vi "CRYView Model LIB.vi"(7 "sAction":string, 8 "nData":i32, 9 "sData":string, 10 "sOption":string, 11 "cView":T1) -> (0 "nData_Out":i32, 1 "sData_Out":string, 3 "cView_Out":T1)   [LabVIEW 2013]
uses:
  CRYView Global.vi
  CRYCurveLibrary/Global/CRYCurve Library Global.vi
  CRYNew View Global.vi
panel:
  out "pSPRef_Out":refnum<vi>
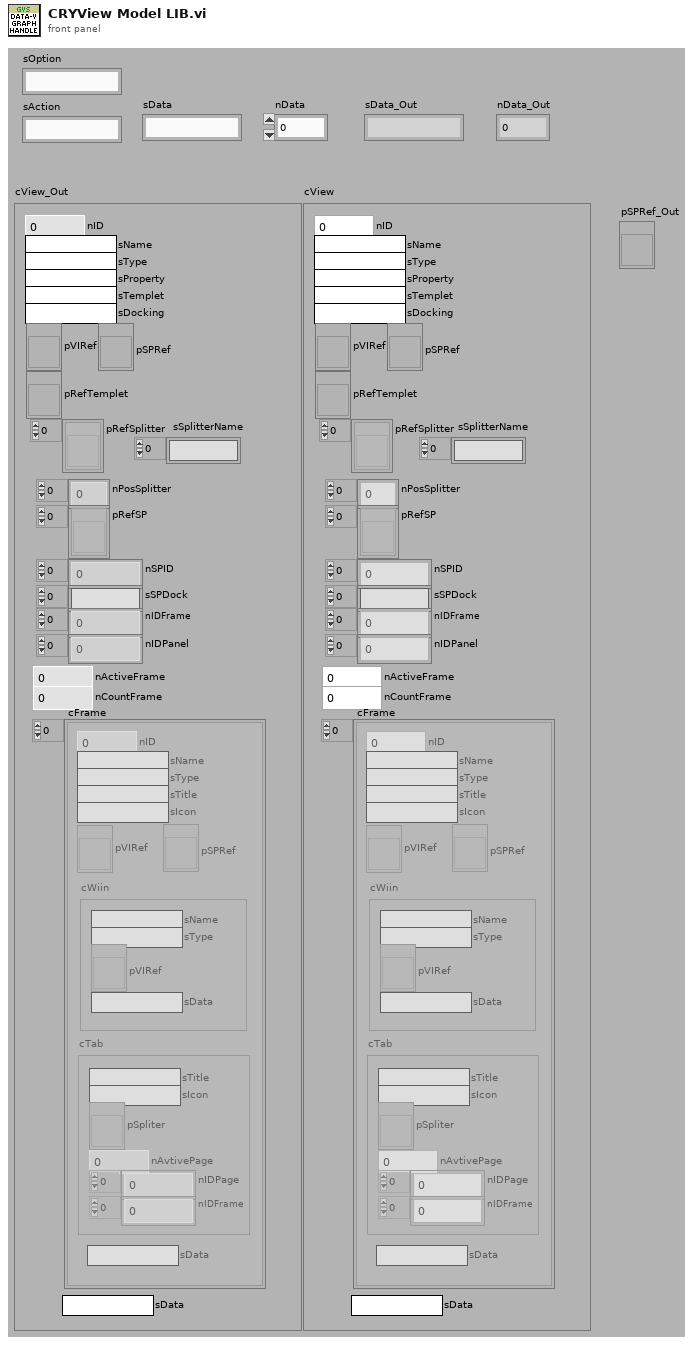
[diagram p1: front panel]
types:
  T1 = cluster{"nID":i32, "sName":string, "sType":string, "sProperty":string, "sTemplet":string, "sDocking":string, "pVIRef":refnum<vi>, "pSPRef":refnum<vi>, "pRefTemplet":refnum<vi>, "pRefSplitter":refnum<vi>[], "nPosSplitter":i32[], "pRefSP":refnum<vi>[], "nSPID":i32[], "sSPDock":string[], "nIDFrame":i32[], "nIDPanel":i32[], "nActiveFrame":i32, "nCountFrame":i32, "cFrame":cluster{"nID":i32, "sName":string, "sType":string, "sTitle":string, "sIcon":string, "pVIRef":refnum<vi>, "pSPRef":refnum<vi>, "cWiin":cluster{"sName":string, "sType":string, "pVIRef":refnum<vi>, "sData":string}, "cTab":cluster{"sTitle":string, "sIcon":string, "pSpliter":refnum<vi>, "nAvtivePage":i32, "nIDPage":i32[], "nIDFrame":i32[]}, "sData":string}[], "sData":string, "sSplitterName":string[]}
  T2 = typedef "Graph Main Info Cluster.ctl" = cluster{"Selected_BarIdx":i32, "Selected_PanelIdx":i32, "Graph Main VIRef":refnum<vi>, "ToolBarClick":bool, "Spliter Ref Array":refnum<vi>[], "Panel Ref Array":refnum<vi>[], "Spliter_matrix":i32[][], "Panel_matrix":i32[][], "child_spliterIdx_matrix":i32[][], "split_pos_matrix":i32[][], "Title State":bool, "sQueueName":string, "Frame nID":i32, "Graph VIRef Array":cluster{"Graph VIRef":refnum<vi>, "Panel Idx":i32, "Frame VIRef":refnum<vi>, "Icon Ring":i32, "Graph Type":string}[], "View Type":string}
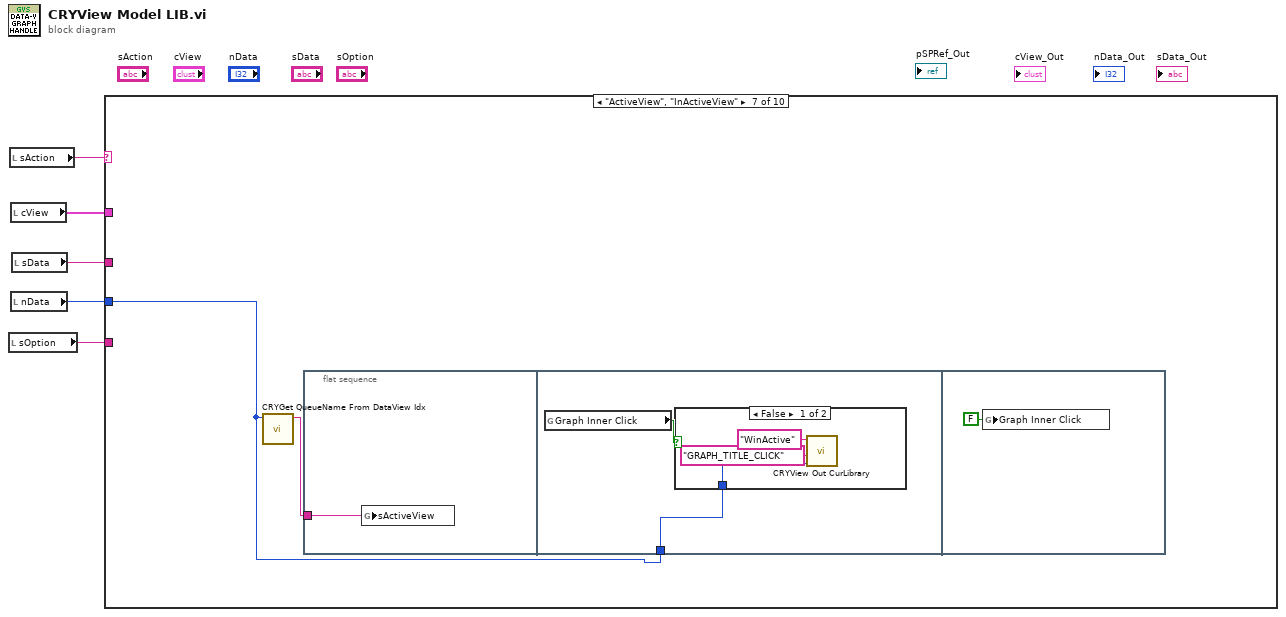
[diagram p0: block diagram]
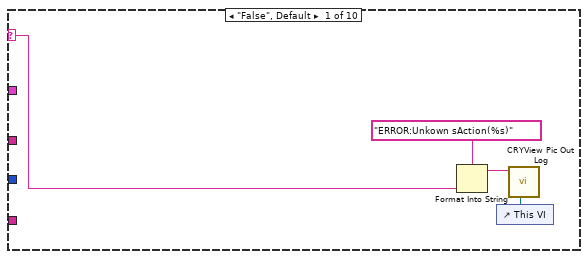
[diagram p2: hidden frame]
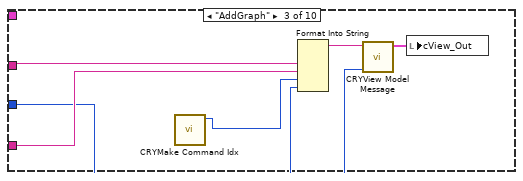
[diagram p4: hidden frame]
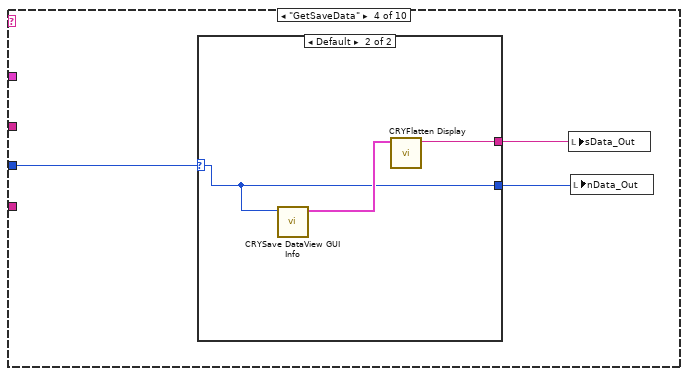
[diagram p5: hidden frame]
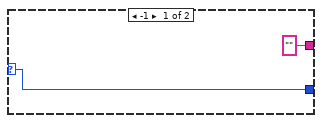
[diagram p6: hidden frame]
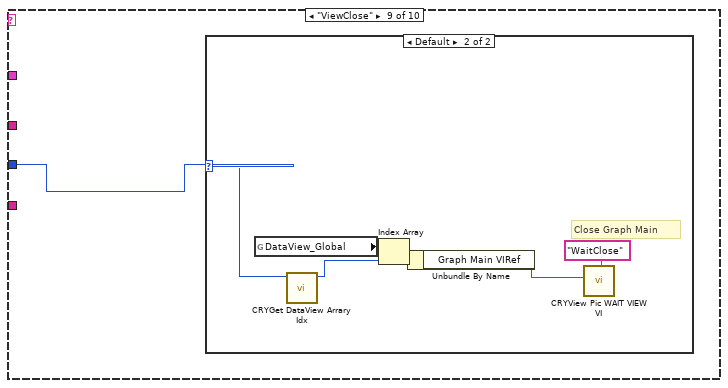
[diagram p11: hidden frame]
diagram:
  n1 = local read "sOption"() -> (w1:string)
  n2 = local read "sAction"() -> (w5:string)
  n3 = local read "cView"() -> (w4:T1)
  n4 = local read "nData"() -> (w2:i32)
  n5 = local read "sData"() -> (w3:string)
  n6 = case shown="\"ActiveView\", \"InActiveView\"" w5 {
    selector: w5 -> [w7 _ _ _ _ _ _ _ _ _]
    tunnel: w4 -> [_ _ _ _ _ _ _ _ _ _]
    tunnel: w3 -> [_ _ w13 _ _ _ _ _ _ _]
    tunnel: w2 -> [_ _ w10 w17 _ _ w25 _ w33 _]
    tunnel: w1 -> [_ _ w12 _ _ _ _ _ _ _]
    frame "False", Default {
      n7 = Format Into String(format string="ERROR:Unkown sAction(%s)", w7) -> (resulting string=w6:string)  [unwired: 2 in, 1 out]
      n8 = control-ref of="This VI"() -> (w9:refnum<vi>)
      n9 = call "CRYView Pic Out Log.vi"("vi reference"=w9, "sData"=w6) -> ()  [unwired: 10 in]
    }
    frame "TitleBarOnOff" {
      # "???????????"
    }
    frame "AddGraph" {
      n10 = call "CRYMake Command Idx.vi"() -> ("New Command Idx"=w14:i32)  [unwired: 11 in]
      n11 = Format Into String(w13, w12, w14, w10) -> (resulting string=w15:string)  [unwired: 3 in, 1 out]
      n12 = call "CRYView Model Message.vi"("nData"=w10, "sMsgData"=w15) -> ("cView_Out"=w11:T1)  [unwired: 7 in, 2 out]
      n13 = local write "cView_Out"(w11) -> ()
    }
    frame "GetSaveData" {
      n14 = case shown="Default" w17 {
        selector: w17 -> [w19 w21]
        tunnel: ["" ("Display flattened") w23] -> w18
        tunnel: [w19 w21] -> w16
        frame -1 {
        }
        frame Default {
          n15 = call "CRYSave DataView GUI Info.vi"("DataView Index"=w21) -> ("DataView GUI Info"=w22:T2)  [unwired: 10 in]
          n16 = call "CRYFlatten Display.vi"("DataView GUI Info"=w22) -> ("Display flattened"=w23:string)  [unwired: 10 in]
        }
      }
      n17 = local write "sData_Out"(w18) -> ()
      n18 = local write "nData_Out"(w16) -> ()
    }
    frame "RemoveView" {
    }
    frame "GetLastView", "GetViewByID" {
    }
    frame "ActiveView", "InActiveView" {
      n19 = call "CRYGet QueueName From DataView Idx.vi"("DataView Idx"=w25) -> ("DataView sQueueName"=w24:string)  [unwired: 10 in]
      n20 = flat-sequence {
        tunnel: w24 -> [w26]
        tunnel: w25 -> [w28]
        frame #0 {
          n21 = global write "CRYView Global.vi" "sActiveView"(w26) -> ()
        }
        frame #1 {
          n22 = global read "CRYCurve Library Global.vi" "Graph Inner Click"() -> (w27:bool)
          n23 = case shown="False" w27 {
            tunnel: w28 -> [w29 _]
            frame False {
              n24 = call "CRYView Out CurLibrary.vi"("DataView Idx"=w29, "sData"="GRAPH_TITLE_CLICK", "sAction"="WinActive") -> ()  [unwired: 7 in, 2 out]
            }
            frame True {
            }
          }
        }
        frame #2 {
          n25 = global write "CRYCurve Library Global.vi" "Graph Inner Click"(FALSE ("Graph Inner Click")) -> ()
        }
      }
    }
    frame "AllInActiveView" {
    }
    frame "ViewClose" {
      n26 = case shown="Default" w33 {
        selector: w33 -> [_ w39]
        frame -1 {
        }
        frame Default {
          # "Close Graph Main"
          n27 = global read "CRYNew View Global.vi" "DataView_Global"() -> (w37:T2[])
          n28 = call "CRYGet DataView Arrary Idx.vi"("DataView Idx In"=w39) -> ("DataView Arrary Idx out"=w35:i32)  [unwired: 10 in]
          n29 = Index Array(array=w37, index=w35) -> (element=w36:T2)
          n30 = Unbundle By Name(w36) -> ("Graph Main VIRef"=w38:refnum<vi>)
          n31 = call "CRYView Pic WAIT VIEW VI.vi"("vi reference"=w38, "sAction"="WaitClose") -> ()  [unwired: 9 in, 1 out]
        }
      }
    }
    frame "ReplaceView" {
    }
  }
